vi "Menu 3 solved.vi"() -> ()   [LabVIEW 2015]
uses:
  <vilib>/Utility/miscctls.llb/LVMenuShortCut.ctl
panel:
  out "Status":bool
  out "Application Status":string
  out "ItemPath":string
  out "ItemTag":string
  in  "stop":bool
  in  "Change menu":bool
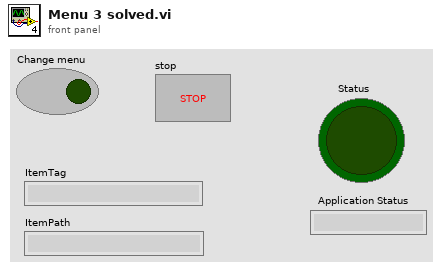
[diagram p1: front panel]
types:
  T1 = typedef "LVMenuShortCut.ctl" = cluster{"Include Shift Key?":bool, "Include Ctrl Key?":bool, "Shortcut Key":string}
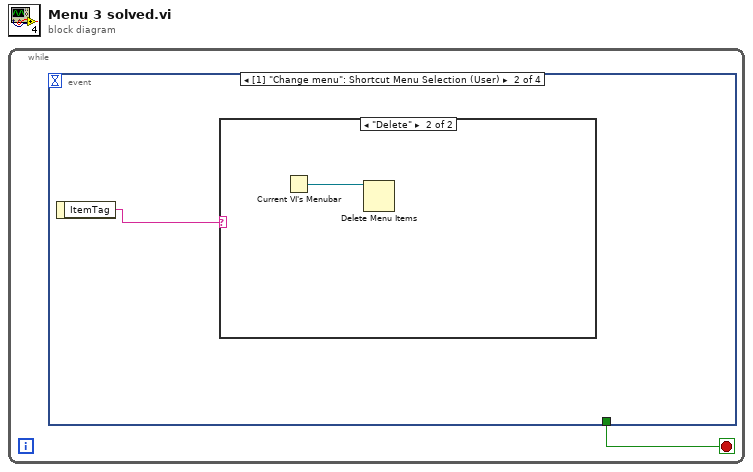
[diagram p0: block diagram]
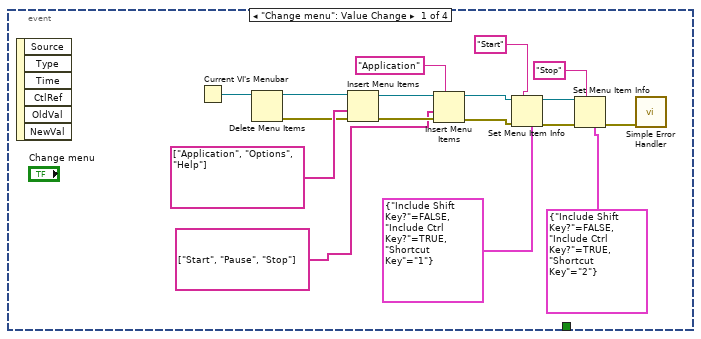
[diagram p2: hidden frame]
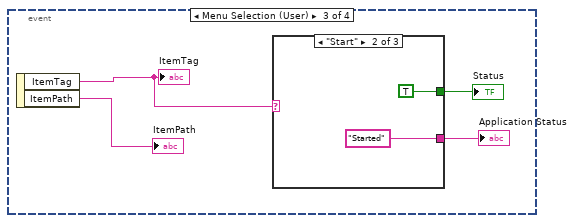
[diagram p4: hidden frame]
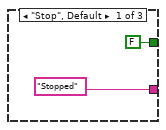
[diagram p5: hidden frame]
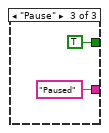
[diagram p6: hidden frame]
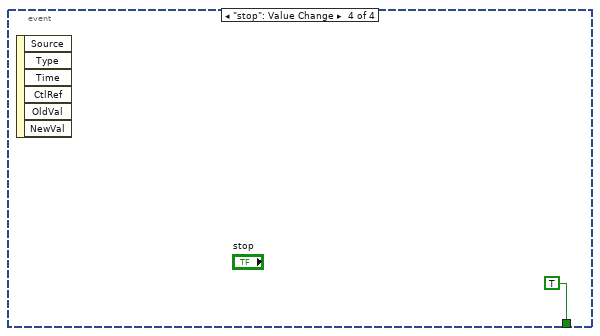
[diagram p7: hidden frame]
diagram:
  n1 = while {
    stop <- w1 stop-if-true
    n2 = event shown="[1] \"Change menu\": Shortcut Menu Selection (User)" {
      selector: _ -> [_ _ _ _]
      dyn-events: _ -> [_ _ _ _]
      timeout: _ -> [_ _ _ _]
      tunnel: [_ _ _ TRUE] -> w1
      event "Change menu": Value Change {
        n3 = event-data() -> ()  [unwired: 1 in, 6 out]
        n4 = Current VI's Menubar() -> (w16:refnum<k9>)
        n5 = Delete Menu Items(9:w16) -> (0:w15:errorcluster, 3:w17:refnum<k9>)  [unwired: 3 in]
        n6 = Insert Menu Items(6:w15, 7:string[] ["Application", "Options", "Help"] ("L10n_item tags 1"), 9:w17) -> (0:w14:errorcluster, 3:w11:refnum<k9>)  [unwired: 3 in, 1 out]
        n7 = Insert Menu Items(5:"Application" ("menu tag"), 6:w14, 7:string[] ["Start", "Pause", "Stop"] ("L10n_item tags 1"), 9:w11) -> (0:w10:errorcluster, 3:w8:refnum<k9>)  [unwired: 2 in, 1 out]
        n8 = Set Menu Item Info(4:T1 {"Include Shift Key?"=FALSE, "Include Ctrl Key?"=TRUE, "Shortcut Key"="1"} ("short cut"), 7:"Start" ("item tag"), 8:w10, 11:w8) -> (0:w6:errorcluster, 3:w2:refnum<k9>)  [unwired: 3 in]
        n9 = Set Menu Item Info(4:T1 {"Include Shift Key?"=FALSE, "Include Ctrl Key?"=TRUE, "Shortcut Key"="2"} ("short cut"), 7:"Stop" ("item tag"), 8:w6, 11:w2) -> (0:w5:errorcluster)  [unwired: 3 in, 1 out]
        n10 = call <vilib>:"Simple Error Handler.vi"("error in (no error)"=w5) -> ()  [unwired: 4 in, 5 out]
      }
      event "Change menu": Shortcut Menu Selection (User) {
        n11 = event-data() -> ("ItemTag"=w19:string)  [unwired: 1 in]
        n12 = case shown="\"Delete\"" w19 {
          frame "False", Default {
          }
          frame "Delete" {
            n13 = Current VI's Menubar() -> (w20:refnum<k9>)
            n14 = Delete Menu Items(9:w20) -> ()  [unwired: 3 in, 2 out]
          }
        }
      }
      event Menu Selection (User) {
        n15 = event-data() -> ("ItemTag"=w23:string, "ItemPath"=→"ItemPath":string)  [unwired: 1 in]
        "ItemTag" <- w23
        n16 = case shown="\"Start\"" w23 {
          tunnel: [FALSE ("Status") TRUE ("Status") TRUE ("Status")] -> w22
          tunnel: ["Stopped" "Started" "Paused"] -> w21
          frame "Stop", Default {
          }
          frame "Start" {
          }
          frame "Pause" {
          }
        }
        "Application Status" <- w21
        "Status" <- w22
      }
      event "stop": Value Change {
        n17 = event-data() -> ()  [unwired: 1 in, 6 out]
      }
    }
  }
